vi "Read Mouse.vi"(2 "Read Address":u8, 3 "Mouse IO":T1) -> (0 "Data out":u8, 1 "Mouse IO Out":T1)   [LabVIEW 2012]
uses:
  <vilib>/rvi/eio/common/nirviEmuTemplateMethod_errors.vi
  <vilib>/eio/EIONode/EIONode.xnode
  <vilib>/eio/EIOMethodNode/EIOMethodNode.xnode
panel:
  out "Array":bool[](array[boolean])
  out "reversed array":bool[](array[boolean])
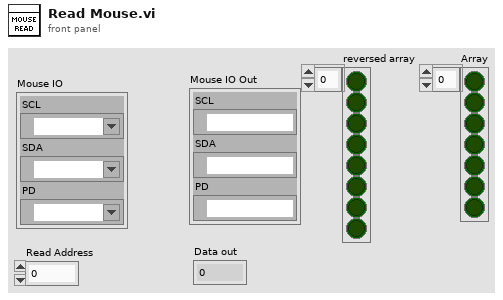
[diagram p1: front panel]
types:
  T1 = cluster{"SCL":refnum<k21>, "SDA":refnum<k21>, "PD":refnum<k21>}
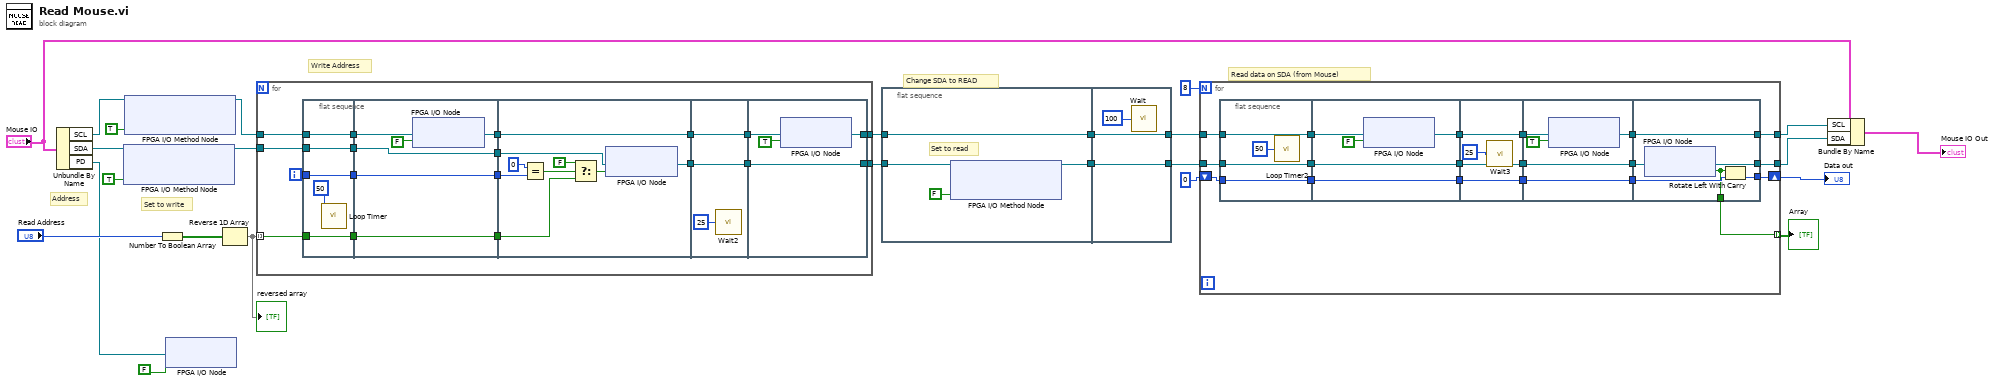
[diagram p0: block diagram]
diagram:
  # "Read data on SDA (from Mouse)"
  # "Change SDA to READ"
  # "Write Address"
  # "Set to write"
  # "Address"
  n1 = Unbundle By Name("Mouse IO") -> ("SCL"=w6:refnum<k21>, "SDA"=w17:refnum<k21>, "PD"=w2:refnum<k21>)
  n2 = xnode "FPGA I/O Method Node"("FPGA I/O In"=w17, "Enable"=TRUE) -> ("FPGA I/O Out"=w16:refnum<k21>)
  n3 = xnode "FPGA I/O Method Node"("FPGA I/O In"=w6, "Enable"=TRUE) -> ("FPGA I/O Out"=w5:refnum<k21>)
  n4 = Number To Boolean Array(number="Read Address") -> (Boolean array=w13:bool[])
  n5 = xnode "FPGA I/O Node"("I/O Item"=FALSE, "FPGA I/O In"=w2) -> ()  [unwired: 1 out]
  n6 = Reverse 1D Array(array=w13) -> (reversed array=w14:bool[])
  "reversed array" <- w14
  n7 = for {
    tunnel: w5 -> [w43]
    tunnel: w16 -> [w40]
    tunnel: w14 -> [w36] mode=indexing
    tunnel: [w35] -> w19
    tunnel: [w34] -> w15
    i -> [w38]
    n8 = flat-sequence {
      tunnel: w36 -> [w45]
      tunnel: w38 -> [w46]
      tunnel: w40 -> [w47]
      tunnel: w43 -> [w48]
      tunnel: [w48] -> w29
      tunnel: [w47] -> w28
      tunnel: [w46] -> w27
      tunnel: [w45] -> w26
      tunnel: [w52] -> w42
      tunnel: [w51] -> w41
      tunnel: [w50] -> w39
      tunnel: [w49] -> w37
      tunnel: w29 -> [w54]
      tunnel: w28 -> [w51]
      tunnel: w27 -> [w50]
      tunnel: w26 -> [w49]
      tunnel: w42 -> [w63]
      tunnel: [w63] -> w33
      tunnel: w41 -> [w62]
      tunnel: w39 -> [w60]
      tunnel: w37 -> [w58]
      tunnel: [w55] -> w31
      tunnel: w33 -> [w66]
      tunnel: [w66] -> w32
      tunnel: w31 -> [w65]
      tunnel: [w65] -> w30
      tunnel: w32 -> [w69]
      tunnel: [w68] -> w35
      tunnel: w30 -> [w67]
      tunnel: [w67] -> w34
      frame #0 {
        n9 = call "Loop Timer"("Count(uSec)"=u16 50) -> ()  [unwired: 1 out]
      }
      frame #1 {
        n10 = xnode "FPGA I/O Node"("I/O Item"=FALSE, "FPGA I/O In"=w54) -> ("FPGA I/O Out"=w52:refnum<k21>)
      }
      frame #2 {
        n11 = Equal?(x=0 ("y"), y=w60) -> (x = y?=w61:bool)
        n12 = Select(t=FALSE, s=w61, f=w58) -> (s? t:f=w56:bool)
        n13 = xnode "FPGA I/O Node"("I/O Item"=w56, "FPGA I/O In"=w62) -> ("FPGA I/O Out"=w55:refnum<k21>)
      }
      frame #3 {
        n14 = call "Wait2"("Count(uSec)"=u16 25) -> ()  [unwired: 1 out]
      }
      frame #4 {
        n15 = xnode "FPGA I/O Node"("I/O Item"=TRUE, "FPGA I/O In"=w69) -> ("FPGA I/O Out"=w68:refnum<k21>)
      }
    }
  }
  n16 = flat-sequence {
    tunnel: w15 -> [w74]
    tunnel: [w72] -> w25
    tunnel: [w71] -> w24
    tunnel: w19 -> [w71]
    tunnel: [w77] -> w21
    tunnel: w25 -> [w77]
    tunnel: w24 -> [w76]
    tunnel: [w76] -> w20
    frame #0 {
      # "Set to read"
      n17 = xnode "FPGA I/O Method Node"("FPGA I/O In"=w74, "Enable"=FALSE) -> ("FPGA I/O Out"=w72:refnum<k21>)
    }
    frame #1 {
      n18 = call "Wait"("Count(uSec)"=u8 100) -> ()  [unwired: 1 out]
    }
  }
  n19 = for {
    N: 8 -> [_]
    tunnel: w20 -> [w96]
    tunnel: w21 -> [w94]
    tunnel: [w93] -> w10
    tunnel: [w91] -> w9
    tunnel: [w78] -> w3 mode=indexing
    shift-right: [w88] -> w11
    shift-left: u8 0 -> [w90]
    n20 = flat-sequence {
      tunnel: w90 -> [w98]
      tunnel: w94 -> [w99]
      tunnel: w96 -> [w100]
      tunnel: [w100] -> w81
      tunnel: [w99] -> w80
      tunnel: [w98] -> w79
      tunnel: [w103] -> w87
      tunnel: [w102] -> w85
      tunnel: [w101] -> w83
      tunnel: w81 -> [w105]
      tunnel: w80 -> [w102]
      tunnel: w79 -> [w101]
      tunnel: w87 -> [w109]
      tunnel: [w109] -> w86
      tunnel: w85 -> [w108]
      tunnel: [w108] -> w84
      tunnel: w83 -> [w107]
      tunnel: [w107] -> w82
      tunnel: w86 -> [w114]
      tunnel: [w113] -> w95
      tunnel: w84 -> [w111]
      tunnel: [w111] -> w92
      tunnel: [w110] -> w89
      tunnel: w82 -> [w110]
      tunnel: w95 -> [w120]
      tunnel: [w120] -> w93
      tunnel: w92 -> [w119]
      tunnel: [w118] -> w91
      tunnel: [w116] -> w88
      tunnel: w89 -> [w117]
      tunnel: [w115] -> w78
      frame #0 {
        n21 = call "Loop Timer2"("Count(uSec)"=u16 50) -> ()  [unwired: 1 out]
      }
      frame #1 {
        n22 = xnode "FPGA I/O Node"("I/O Item"=FALSE, "FPGA I/O In"=w105) -> ("FPGA I/O Out"=w103:refnum<k21>)
      }
      frame #2 {
        n23 = call "Wait3"("Count(uSec)"=u8 25) -> ()  [unwired: 1 out]
      }
      frame #3 {
        n24 = xnode "FPGA I/O Node"("I/O Item"=TRUE, "FPGA I/O In"=w114) -> ("FPGA I/O Out"=w113:refnum<k21>)
      }
      frame #4 {
        n25 = xnode "FPGA I/O Node"("FPGA I/O In"=w119) -> ("I/O Item"=w115:bool, "FPGA I/O Out"=w118:refnum<k21>)
        n26 = Rotate Left With Carry(2:w117, 3:w115) -> (0:w116:u8)  [unwired: 1 out]
      }
    }
  }
  "Data out" <- w11
  "Array" <- w3
  n27 = Bundle By Name(cluster="Mouse IO", "SCL"=w10, "SDA"=w9) -> (→"Mouse IO Out":T1)
